vi "this_vis_ref.vi"() -> (7 "vi ref":refnum<vi>)   [LabVIEW 2015]
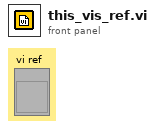
[diagram p1: front panel]
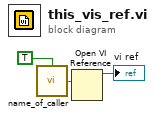
[diagram p0: block diagram]
diagram:
  n1 = call "name_of_caller.vi"("is in inlined vi? (F)"=TRUE) -> ("name of caller out"=w2:string)  [unwired: 3 in]
  n2 = Open VI Reference(vi path=w2) -> (vi reference=→"vi ref":refnum<vi>)  [unwired: 5 in, 1 out]
